vi "Send Send Software Trigger.vi"(7 "Message Priority (Normal)":T1=enum."Normal", 8 "error in (no error)":errorcluster, 10 "Execute?":bool, 11 "Message Enqueuer":refnum<class "Message Enqueuer.lvclass">) -> (0 "error out":errorcluster, 3 "Message Enqueuer out":refnum<class "Message Enqueuer.lvclass">)   [LabVIEW 2016, in "CS++DMM.lvlib" / "Send Software Trigger Msg.lvclass"]
doc: "Sends the <B>CS++DMM.lvlib:Send Software Trigger Msg.lvclass</B> message.\n\n<B>CS++DMM.lvlib:CS++DMM.lvclass:Send Software Trigger.vi</B> Description:\n\nThis VI sends a command to trigger the DMM. Call this VI if you pass IVIDMM_VAL_SOFTWARE_TRIG for the Trigger Source parameter of the Configure Trigger VI or the Sample Trigger parameter of the Configure Multi-Point [MP] VI.\n\nNotes:\n\n(1) This VI is part of the IviDmmSoftwareTrigger [SWT] extension group.\n\n(2) If neither the IviDmm>Trigger>Trigger Source nor the IviDmm>Multi-Point Acquisition>Sample Trigger [MP] property is set to the IVIDMM_VAL_SOFTWARE_TRIG value, this VI returns an error.\n\n(3) This VI does not check the instrument status. Typically, you call this VI only in a sequence of calls to other low-level driver VIs. The sequence performs one operation. You use the low-level VIs to optimize one or more aspects of interaction with the instrument. If you want to check the instrument status, call the Error-Query VI at the conclusion of the sequence."
uses:
  Send Software Trigger Msg.lvclass
  <vilib>/ActorFramework/Message Enqueuer/Message Enqueuer.lvclass
  <vilib>/ActorFramework/Message Enqueuer/Message Priority.ctl
  C:/Program Files (x86)/National Instruments/LabVIEW 2016/vi.lib/ActorFramework/Message/Message.lvclass
  Send Software Trigger Msg.lvclass/Send Software Trigger Msg.ctl
  <vilib>/ActorFramework/Message Enqueuer/Message Enqueuer.lvclass/Message Enqueuer.ctl
  <vilib>/ActorFramework/Message Priority Queue/Priority Enqueue.vi
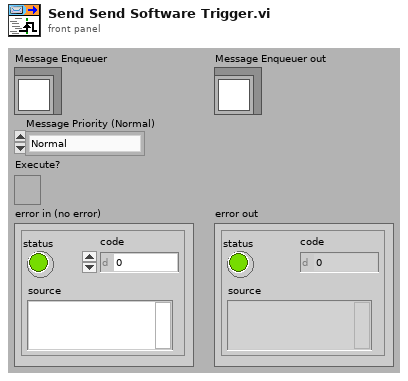
[diagram p1: front panel]
types:
  T1 = typedef "Actor Framework.lvlib/Message Enqueuer.lvclass/Message Priority.ctl" = enum16{"Low", "Normal", "High"}
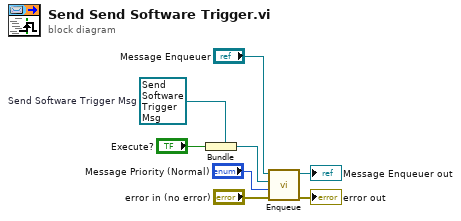
[diagram p0: block diagram]
diagram:
  w2 = refnum<class "Send Software Trigger Msg.lvclass"> refnum  # Send Software Trigger Msg
  n1 = Bundle(cluster=w2, "Execute?") -> (w5:refnum<class "Send Software Trigger Msg.lvclass">)
  n2 = call <vilib>:"Enqueue.vi"("error in (no error)"="error in (no error)", "Message Priority (Normal)"="Message Priority (Normal)", "Message"=w5, "Message Enqueuer in"="Message Enqueuer") -> ("error out"=→"error out":errorcluster, "Message Enqueuer out"=→"Message Enqueuer out":refnum<class "Message Enqueuer.lvclass">)  [unwired: 6 in]
